vi "Go.vi"(9 "Timing Data":T1(array[cluster]), 10 "Control In":T2={"I-O.lvclass"=refnum, "Gantry"=refnum, "Dispenser"="COM1"}, 11 "Sensor Dispense in":refnum<class "Sensor Dispense.lvclass">) -> (2 "Control Out":T2={"I-O.lvclass"=refnum, "Gantry"=refnum, "Dispenser"="COM1"}, 3 "Sensor Dispense out":refnum<class "Sensor Dispense.lvclass">)   [LabVIEW 2021, in "Sensor Dispense.lvclass"]
uses:
  Sensor Dispense.lvclass
  C:/Users/HEP/Documents/GitHub/UCSB-Gantry-HEP/Classes/Routine/Dispense/Dispense.lvclass
  Classes/Controller/Controllers.ctl
  Classes/Controller/I-O/I-O.lvclass
  C:/Program Files (x86)/Aerotech/A3200/LabVIEW/2010/Bin/Aerotech.A3200.dll
  Program Files (x86)/Aerotech/A3200/LabVIEW/2010/Bin/Aerotech.A3200.dll
  Sensor Dispense.lvclass/Sensor Dispense.ctl
  Classes/Controller/Motion/Motion.lvclass
  Classes/Controller/Dispenser/Dispenser.lvclass
  Classes/Controller/Motion/A3200/A3200.lvclass
  Classes/Controller/Controller.lvclass
panel:
  out "error out":errorcluster
  in  "error in (no error)":errorcluster
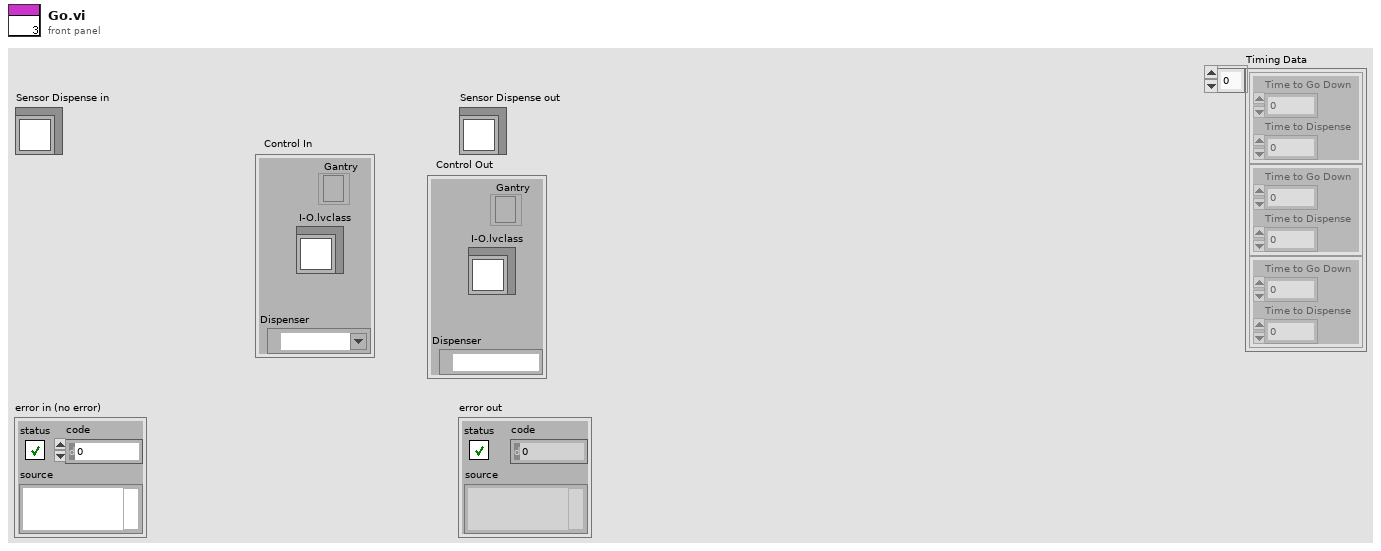
[diagram p1: front panel]
types:
  T1 = cluster{"Time to Go Down":i32, "Time to Dispense":i32}[]
  T2 = typedef "Controller.lvclass/Controllers.ctl" = cluster{"I-O.lvclass":refnum<class "I-O.lvclass">, "Gantry":refnum<k24>, "Dispenser":refnum<visa-resource-name>}
  T3 = cluster{"Endpoints":dbl[][], "Center":dbl[], "CW/CCW":dbl, "Dispense Type":enum16{"N-gon", "Square", "Arc", "Dot", "Line", "Circle"}}[]
  T4 = enum16{"N-gon", "Square", "Arc", "Dot", "Line", "Circle"}
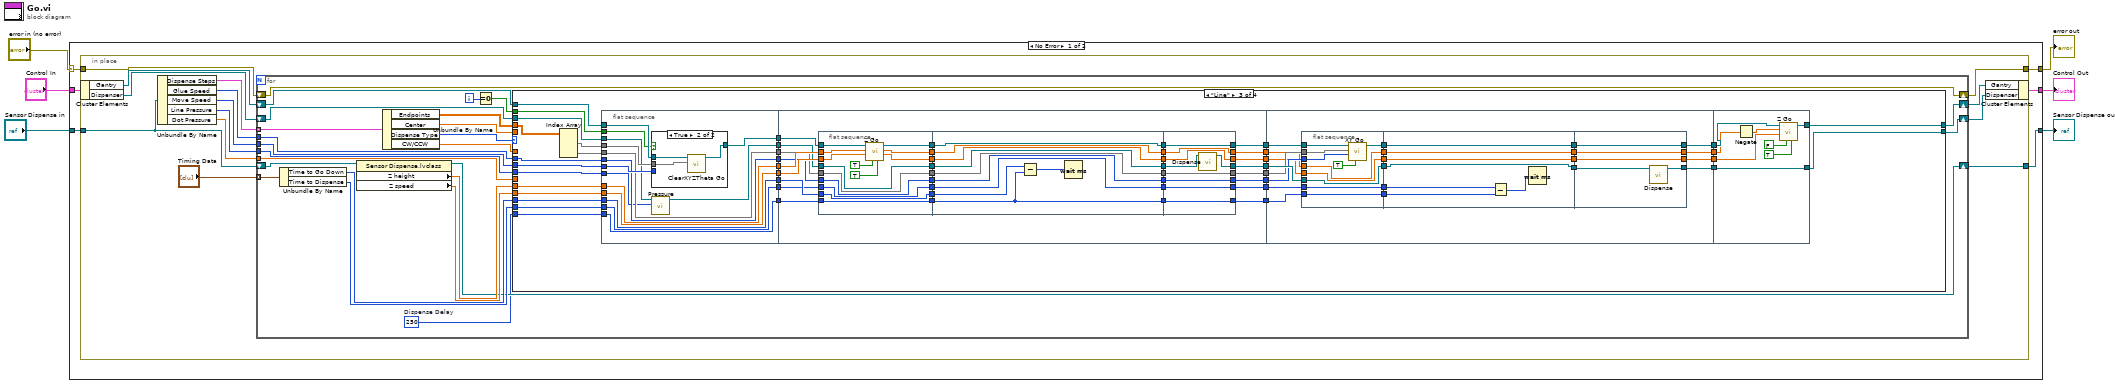
[diagram p0: block diagram]
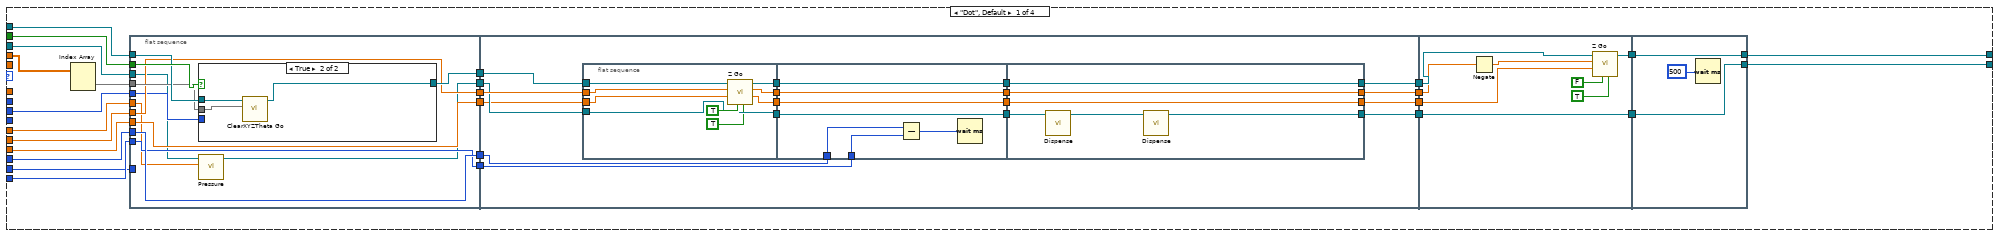
[diagram p2: hidden frame]
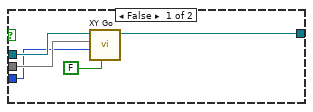
[diagram p3: hidden frame]
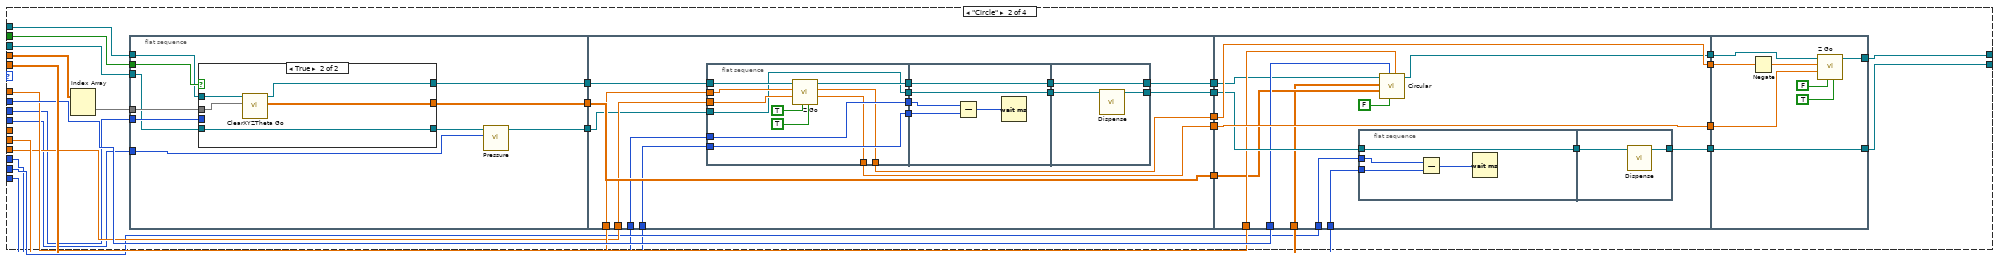
[diagram p4: hidden frame]
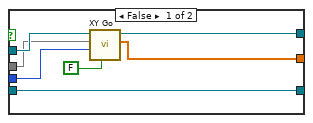
[diagram p5: hidden frame]
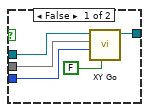
[diagram p6: hidden frame]
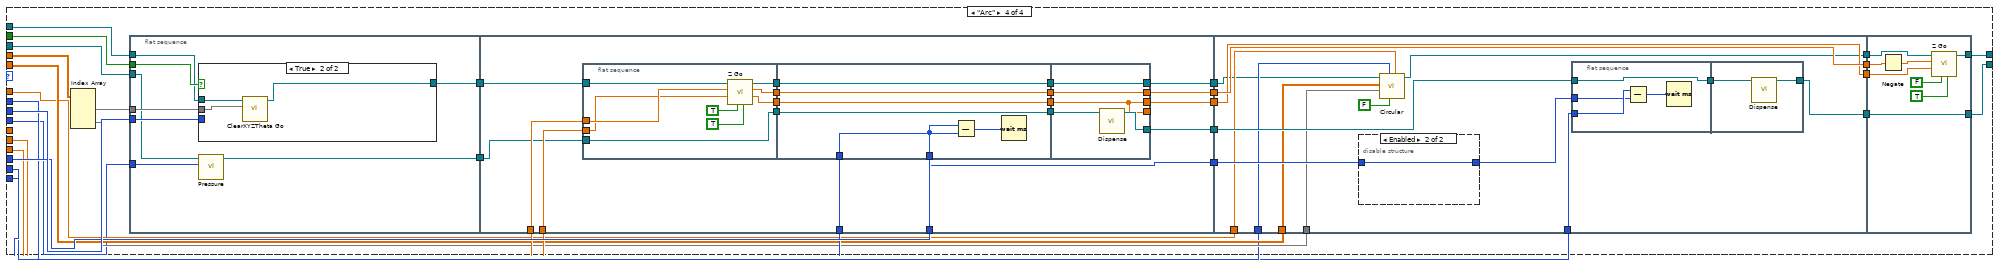
[diagram p7: hidden frame]
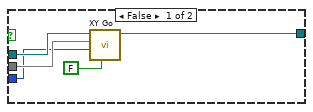
[diagram p8: hidden frame]
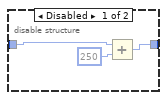
[diagram p9: hidden frame]
diagram:
  n1 = case shown="No Error" "error in (no error)" {
    selector: "error in (no error)" -> [w7 w562]
    tunnel: "Sensor Dispense in" -> [w12 w561]
    tunnel: [w11 w561] -> w5
    tunnel: "Control In" -> [w10 w560]
    tunnel: [w9 w560] -> w3
    tunnel: [w8 w562] -> w2
    frame No Error {
      n2 = in-place {
        in-place-border: w12 -> [w24]
        in-place-border: [w23] -> w11
        in-place-border: w7 -> [w17]
        in-place-border: [w16] -> w8
        n3 = in-place-cluster #1(w10) -> ("Gantry"=w25:refnum<k24>, "Dispenser"=w20:refnum<visa-resource-name>)
        n4 = Unbundle By Name(w24) -> ("Dispense Steps"=w21:T3, "Glue Speed"=w15:i32, "Move Speed"=w26:i32, "Line Pressure"=w13:i64, "Dot Pressure"=w14:dbl)
        n5 = for {
          tunnel: w26 -> [w50]
          shift-right: [w41] -> w22
          shift-left: w25 -> [w48]
          tunnel: w15 -> [w49]
          shift-right: [w32] -> w23
          shift-left: w24 -> [w46]
          tunnel: w21 -> [w43] mode=indexing
          shift-right: [w36] -> w18
          shift-left: w20 -> [w39]
          tunnel: "Timing Data" -> [w38] mode=indexing
          shift-right: [w27] -> w16
          shift-left: w17 -> [w27]
          tunnel: w14 -> [w29]
          tunnel: w13 -> [w28]
          i -> [w45]
          w31 = 250  # Dispense Delay
          n6 = Unbundle By Name(w38) -> ("Time to Go Down"=w37:i32, "Time to Dispense"=w33:i32)
          n7 = property class="Sensor Dispense.lvclass"(reference=w46) -> (reference out=w32:refnum<class "Sensor Dispense.lvclass">, "Z height"=w35:dbl, "Z speed"=w34:dbl)  [unwired: 1 in, 1 out]
          n8 = Unbundle By Name(w43) -> ("Endpoints"=w30:dbl[][], "Center"=w40:dbl[], "Dispense Type"=w42:T4, "CW/CCW"=w47:dbl)
          n9 = Equal To 0?(x=w45) -> (x = 0?=w44:bool)
          n10 = case shown="\"Line\"" w42 {
            tunnel: w40 -> [_ w172 _ w452]
            tunnel: w48 -> [w75 w173 w299 w461]
            tunnel: w50 -> [w58 w166 w298 w458]
            tunnel: [w74 w176 w295 w447] -> w41
            tunnel: w49 -> [_ w171 w285 w451]
            tunnel: w47 -> [_ w170 _ w450]
            tunnel: w34 -> [w66 w168 w282 w454]
            tunnel: w35 -> [w67 w169 w283 w455]
            tunnel: w44 -> [w76 w167 w297 w462]
            tunnel: w39 -> [w65 w150 w289 w443]
            tunnel: w37 -> [w63 w157 w287 w457]
            tunnel: w33 -> [w68 w158 w284 w449]
            tunnel: w31 -> [w69 w156 w288 w456]
            tunnel: [w73 w151 w292 w446] -> w36
            tunnel: w30 -> [w72 w155 w291 w460]
            tunnel: w29 -> [w57 _ _ _]
            tunnel: w28 -> [_ w148 w263 w442]
            frame "Dot", Default {
              n11 = Index Array(array=w72) -> (element=w71:dbl[])  [unwired: 2 in]
              n12 = flat-sequence {
                tunnel: w76 -> [w88]
                tunnel: w75 -> [w87]
                tunnel: w71 -> [w86]
                tunnel: [w85] -> w70
                tunnel: w69 -> [w82]
                tunnel: w68 -> [_]
                tunnel: w67 -> [w84]
                tunnel: w66 -> [w81]
                tunnel: w65 -> [w79]
                tunnel: [w84] -> w64
                tunnel: w63 -> [w83]
                tunnel: [w83] -> w62
                tunnel: [w82] -> w61
                tunnel: [w78] -> w60
                tunnel: [w81] -> w59
                tunnel: w58 -> [w80]
                tunnel: w57 -> [w77]
                tunnel: [w114] -> w54
                tunnel: w70 -> [w113]
                tunnel: [w110] -> w53
                tunnel: w64 -> [w109]
                tunnel: w62 -> [w108]
                tunnel: w61 -> [w107]
                tunnel: w60 -> [w106]
                tunnel: w59 -> [w103]
                tunnel: [w100] -> w52
                tunnel: [w99] -> w51
                tunnel: w54 -> [w142]
                tunnel: w53 -> [w141]
                tunnel: w52 -> [w140]
                tunnel: w51 -> [w139]
                tunnel: [w143] -> w56
                tunnel: [w142] -> w55
                tunnel: [w146] -> w73
                tunnel: [w147] -> w74
                tunnel: w56 -> [w147]
                tunnel: w55 -> [w146]
                frame #0 {
                  n13 = case shown="True" w88 {
                    tunnel: w87 -> [w93 w96]
                    tunnel: [w92 w95] -> w85
                    tunnel: w86 -> [w91 w94]
                    tunnel: w80 -> [w90 _]
                    frame False {
                      n14 = call "XY Go.vi"("return immediately"=FALSE, "Speed"=w90, "XY In"=w91, "Gantry In"=w93) -> ("Gantry Out"=w92:refnum<k24>)  [unwired: 5 in, 2 out]
                    }
                    frame True {
                      n15 = call "ClearXYZTheta Go.vi"("XYZTheta In"=w94, "Gantry In"=w96) -> ("Gantry Out"=w95:refnum<k24>)  [unwired: 7 in, 2 out]
                    }
                  }
                  n16 = call "Pressure.vi"("Pressure"=w77, "VISA resource name"=w79) -> ("VISA resource name out"=w78:refnum<visa-resource-name>)  [unwired: 8 in, 1 out]
                }
                frame #1 {
                  n17 = flat-sequence {
                    tunnel: w113 -> [w123]
                    tunnel: [w122] -> w111
                    tunnel: w109 -> [w121]
                    tunnel: w106 -> [w119]
                    tunnel: [w119] -> w105
                    tunnel: w103 -> [w118]
                    tunnel: [w117] -> w102
                    tunnel: [w116] -> w97
                    tunnel: [w129] -> w112
                    tunnel: w111 -> [w129]
                    tunnel: w108 -> [w128]
                    tunnel: w107 -> [w127]
                    tunnel: w105 -> [w126]
                    tunnel: [w126] -> w104
                    tunnel: w102 -> [w125]
                    tunnel: [w125] -> w101
                    tunnel: [w124] -> w98
                    tunnel: w97 -> [w124]
                    tunnel: [w136] -> w114
                    tunnel: w112 -> [w135]
                    tunnel: [w135] -> w110
                    tunnel: w104 -> [w134]
                    tunnel: w101 -> [w132]
                    tunnel: [w132] -> w100
                    tunnel: [w131] -> w99
                    tunnel: w98 -> [w131]
                    frame #0 {
                      n18 = call "Z Go.vi"("Increment"=TRUE, "Return Immediately"=TRUE, "Speed In"=w118, "Position In"=w121, "Gantry In"=w123) -> ("Speed Out"=w116:dbl, "Position Out"=w117:dbl, "Gantry Out"=w122:refnum<k24>)  [unwired: 3 in, 1 out]
                    }
                    frame #1 {
                      n19 = Subtract(x=w128, y=w127) -> (x-y=w130:i32)
                      n20 = Wait (ms)(milliseconds to wait=w130) -> ()  [unwired: 1 out]
                    }
                    frame #2 {
                      n21 = call "Dispense.vi"("Dispenser In"=w134) -> ("Dispenser Out"=w133:refnum<visa-resource-name>)  [unwired: 9 in, 1 out]
                      n22 = call "Dispense.vi"("Dispenser In"=w133) -> ("Dispenser Out"=w136:refnum<visa-resource-name>)  [unwired: 9 in, 1 out]
                    }
                  }
                }
                frame #2 {
                  n23 = Negate(x=w140) -> (-x=w144:dbl)
                  n24 = call "Z Go.vi"("Increment"=TRUE, "Return Immediately"=FALSE, "Speed In"=w139, "Position In"=w144, "Gantry In"=w141) -> ("Gantry Out"=w143:refnum<k24>)  [unwired: 3 in, 3 out]
                }
                frame #3 {
                  n25 = Wait (ms)(milliseconds to wait=u32 500) -> ()  [unwired: 1 out]
                }
              }
            }
            frame "Circle" {
              n26 = Index Array(array=w155) -> (element=w154:dbl[])  [unwired: 2 in]
              n27 = flat-sequence {
                tunnel: [w184] -> w175
                tunnel: w173 -> [w185]
                tunnel: w167 -> [w186]
                tunnel: w166 -> [w183]
                tunnel: [w182] -> w164
                tunnel: w154 -> [w181]
                tunnel: w150 -> [w180]
                tunnel: [w178] -> w149
                tunnel: w148 -> [w177]
                tunnel: w169 -> [w208]
                tunnel: w168 -> [w209]
                tunnel: [w215] -> w165
                tunnel: [w206] -> w163
                tunnel: [w207] -> w162
                tunnel: w164 -> [w215]
                tunnel: w175 -> [w205]
                tunnel: [w214] -> w159
                tunnel: w157 -> [w213]
                tunnel: w156 -> [w212]
                tunnel: [w202] -> w153
                tunnel: w149 -> [w201]
                tunnel: [w235] -> w174
                tunnel: [w248] -> w161
                tunnel: [w247] -> w160
                tunnel: w156 -> [w245]
                tunnel: w158 -> [w246]
                tunnel: w159 -> [w243]
                tunnel: w165 -> [w238]
                tunnel: w163 -> [w248]
                tunnel: w162 -> [w247]
                tunnel: w170 -> [w241]
                tunnel: w171 -> [w239]
                tunnel: w172 -> [w237]
                tunnel: w153 -> [w236]
                tunnel: [w244] -> w152
                tunnel: [w260] -> w176
                tunnel: w174 -> [w261]
                tunnel: w161 -> [w262]
                tunnel: w160 -> [w259]
                tunnel: w152 -> [w258]
                tunnel: [w258] -> w151
                frame #0 {
                  n28 = case shown="True" w186 {
                    tunnel: w185 -> [w193 w198]
                    tunnel: [w192 w197] -> w184
                    tunnel: w183 -> [w191 _]
                    tunnel: [w190 w195] -> w182
                    tunnel: w181 -> [w189 w196]
                    tunnel: w180 -> [w188 w194]
                    tunnel: [w188 w194] -> w179
                    frame False {
                      n29 = call "XY Go.vi"("return immediately"=FALSE, "Speed"=w191, "XY In"=w189, "Gantry In"=w193) -> ("XY Out"=w190:dbl[], "Gantry Out"=w192:refnum<k24>)  [unwired: 5 in, 1 out]
                    }
                    frame True {
                      n30 = call "ClearXYZTheta Go.vi"("XYZTheta In"=w196, "Gantry In"=w198) -> ("XYZTheta Out"=w195:dbl[], "Gantry Out"=w197:refnum<k24>)  [unwired: 7 in, 1 out]
                    }
                  }
                  n31 = call "Pressure.vi"("Pressure"=w177, "VISA resource name"=w179) -> ("VISA resource name out"=w178:refnum<visa-resource-name>)  [unwired: 8 in, 1 out]
                }
                frame #1 {
                  n32 = flat-sequence {
                    tunnel: w212 -> [w225]
                    tunnel: w213 -> [w226]
                    tunnel: [w226] -> w211
                    tunnel: [w225] -> w210
                    tunnel: w209 -> [w224]
                    tunnel: w208 -> [w223]
                    tunnel: [w222] -> w207
                    tunnel: [w221] -> w206
                    tunnel: w205 -> [w220]
                    tunnel: [w219] -> w204
                    tunnel: w201 -> [w217]
                    tunnel: [w217] -> w200
                    tunnel: w211 -> [w230]
                    tunnel: w210 -> [w229]
                    tunnel: w204 -> [w228]
                    tunnel: [w228] -> w203
                    tunnel: w200 -> [w227]
                    tunnel: [w227] -> w199
                    tunnel: [w234] -> w214
                    tunnel: w203 -> [w233]
                    tunnel: [w233] -> w202
                    tunnel: w199 -> [w232]
                    frame #0 {
                      n33 = call "Z Go.vi"("Increment"=TRUE, "Return Immediately"=TRUE ("return immediately"), "Speed In"=w224, "Position In"=w223, "Gantry In"=w220) -> ("Speed Out"=w222:dbl, "Position Out"=w221:dbl, "Gantry Out"=w219:refnum<k24>)  [unwired: 3 in, 1 out]
                    }
                    frame #1 {
                      n34 = Subtract(x=w230, y=w229) -> (x-y=w231:i32)
                      n35 = Wait (ms)(milliseconds to wait=w231) -> ()  [unwired: 1 out]
                    }
                    frame #2 {
                      n36 = call "Dispense.vi"("Dispenser In"=w232) -> ("Dispenser Out"=w234:refnum<visa-resource-name>)  [unwired: 9 in, 1 out]
                    }
                  }
                }
                frame #2 {
                  n37 = flat-sequence {
                    tunnel: [w249] -> w242
                    tunnel: w246 -> [w252]
                    tunnel: w245 -> [w251]
                    tunnel: w243 -> [w249]
                    tunnel: [w254] -> w244
                    tunnel: w242 -> [w253]
                    frame #0 {
                      n38 = Subtract(x=w252, y=w251) -> (x-y=w250:i32)
                      n39 = Wait (ms)(milliseconds to wait=w250) -> ()  [unwired: 1 out]
                    }
                    frame #1 {
                      n40 = call "Dispense.vi"("Dispenser In"=w253) -> ("Dispenser Out"=w254:refnum<visa-resource-name>)  [unwired: 9 in, 1 out]
                    }
                  }
                  n41 = call "Circular.vi"("Direction"=w241, "return immediately"=FALSE, "Speed"=w239, "XY End"=w238, "XY Center"=w237, "Gantry In"=w236) -> ("Gantry Out"=w235:refnum<k24>)  [unwired: 4 in, 1 out]
                }
                frame #3 {
                  n42 = Negate(x=w262) -> (-x=w257:dbl)
                  n43 = call "Z Go.vi"("Increment"=TRUE, "Return Immediately"=FALSE, "Speed In"=w259, "Position In"=w257, "Gantry In"=w261) -> ("Gantry Out"=w260:refnum<k24>)  [unwired: 3 in, 3 out]
                }
              }
            }
            frame "Line" {
              n44 = Index Array(array=w291) -> (element #1=w290:dbl[], element #2=w286:dbl[])  [unwired: 4 in]
              n45 = flat-sequence {
                tunnel: w299 -> [w314]
                tunnel: w298 -> [w313]
                tunnel: w297 -> [w312]
                tunnel: [w311] -> w296
                tunnel: w290 -> [w310]
                tunnel: w289 -> [w302]
                tunnel: w288 -> [w306]
                tunnel: w287 -> [w307]
                tunnel: w286 -> [w305]
                tunnel: w285 -> [w304]
                tunnel: w284 -> [w303]
                tunnel: w283 -> [w309]
                tunnel: w282 -> [w308]
                tunnel: [w309] -> w281
                tunnel: [w308] -> w280
                tunnel: [w307] -> w278
                tunnel: [w306] -> w277
                tunnel: [w301] -> w276
                tunnel: [w305] -> w274
                tunnel: [w304] -> w272
                tunnel: [w303] -> w270
                tunnel: w263 -> [w300]
                tunnel: w296 -> [w355]
                tunnel: [w356] -> w294
                tunnel: w281 -> [w354]
                tunnel: w280 -> [w353]
                tunnel: [w350] -> w279
                tunnel: w278 -> [w348]
                tunnel: w277 -> [w346]
                tunnel: w276 -> [w343]
                tunnel: [w342] -> w275
                tunnel: w274 -> [w339]
                tunnel: [w338] -> w273
                tunnel: w272 -> [w335]
                tunnel: [w331] -> w271
                tunnel: w270 -> [w332]
                tunnel: [w330] -> w269
                tunnel: [w328] -> w266
                tunnel: [w325] -> w264
                tunnel: w294 -> [w407]
                tunnel: [w411] -> w293
                tunnel: w279 -> [w410]
                tunnel: w275 -> [w406]
                tunnel: w273 -> [w405]
                tunnel: w271 -> [w402]
                tunnel: w269 -> [w400]
                tunnel: [w398] -> w268
                tunnel: [w397] -> w267
                tunnel: w266 -> [w394]
                tunnel: [w393] -> w265
                tunnel: w264 -> [w390]
                tunnel: [w441] -> w295
                tunnel: w293 -> [w440]
                tunnel: [w440] -> w292
                tunnel: w268 -> [w439]
                tunnel: w267 -> [w438]
                tunnel: w265 -> [w436]
                frame #0 {
                  n46 = case shown="True" w312 {
                    tunnel: w314 -> [w319 w322]
                    tunnel: w313 -> [w318 _]
                    tunnel: [w317 w321] -> w311
                    tunnel: w310 -> [w316 w320]
                    frame False {
                      n47 = call "XY Go.vi"("return immediately"=FALSE, "Speed"=w318, "XY In"=w316, "Gantry In"=w319) -> ("Gantry Out"=w317:refnum<k24>)  [unwired: 5 in, 2 out]
                    }
                    frame True {
                      n48 = call "ClearXYZTheta Go.vi"("XYZTheta In"=w320, "Gantry In"=w322) -> ("Gantry Out"=w321:refnum<k24>)  [unwired: 7 in, 2 out]
                    }
                  }
                  n49 = call "Pressure.vi"("Pressure"=w300, "VISA resource name"=w302) -> ("VISA resource name out"=w301:refnum<visa-resource-name>)  [unwired: 8 in, 1 out]
                }
                frame #1 {
                  n50 = flat-sequence {
                    tunnel: w355 -> [w370]
                    tunnel: w354 -> [w369]
                    tunnel: w353 -> [w368]
                    tunnel: [w366] -> w352
                    tunnel: [w365] -> w349
                    tunnel: w348 -> [w365]
                    tunnel: [w364] -> w347
                    tunnel: w346 -> [w364]
                    tunnel: [w363] -> w344
                    tunnel: w343 -> [w363]
                    tunnel: [w362] -> w340
                    tunnel: w339 -> [w362]
                    tunnel: [w361] -> w336
                    tunnel: w335 -> [w361]
                    tunnel: [w360] -> w333
                    tunnel: w332 -> [w360]
                    tunnel: [w359] -> w326
                    tunnel: [w358] -> w323
                    tunnel: w352 -> [w379]
                    tunnel: [w379] -> w351
                    tunnel: w349 -> [w378]
                    tunnel: w347 -> [w373]
                    tunnel: [w377] -> w345
                    tunnel: w344 -> [w377]
                    tunnel: [w376] -> w341
                    tunnel: w340 -> [w376]
                    tunnel: [w375] -> w337
                    tunnel: w336 -> [w375]
                    tunnel: [w374] -> w334
                    tunnel: w333 -> [w374]
                    tunnel: [w373] -> w329
                    tunnel: [w372] -> w327
                    tunnel: w326 -> [w372]
                    tunnel: [w371] -> w324
                    tunnel: w323 -> [w371]
                    tunnel: [w389] -> w356
                    tunnel: w351 -> [w388]
                    tunnel: [w388] -> w350
                    tunnel: w345 -> [w383]
                    tunnel: [w387] -> w342
                    tunnel: w341 -> [w387]
                    tunnel: [w386] -> w338
                    tunnel: w337 -> [w386]
                    tunnel: w334 -> [w385]
                    tunnel: [w385] -> w331
                    tunnel: [w384] -> w330
                    tunnel: w329 -> [w384]
                    tunnel: [w382] -> w328
                    tunnel: w327 -> [w382]
                    tunnel: [w381] -> w325
                    tunnel: w324 -> [w381]
                    frame #0 {
                      n51 = call "Z Go.vi"("Increment"=TRUE, "Return Immediately"=TRUE, "Speed In"=w368, "Position In"=w369, "Gantry In"=w370) -> ("Speed Out"=w358:dbl, "Position Out"=w359:dbl, "Gantry Out"=w366:refnum<k24>)  [unwired: 3 in, 1 out]
                    }
                    frame #1 {
                      n52 = Subtract(x=w378, y=w373) -> (x-y=w380:i32)
                      n53 = Wait (ms)(milliseconds to wait=w380) -> ()  [unwired: 1 out]
                    }
                    frame #2 {
                      n54 = call "Dispense.vi"("Dispenser In"=w383) -> ("Dispenser Out"=w389:refnum<visa-resource-name>)  [unwired: 9 in, 1 out]
                    }
                  }
                }
                frame #2 {
                  n55 = flat-sequence {
                    tunnel: w410 -> [w420]
                    tunnel: [w419] -> w408
                    tunnel: w407 -> [w419]
                    tunnel: w406 -> [w418]
                    tunnel: w405 -> [w417]
                    tunnel: [w416] -> w404
                    tunnel: [w415] -> w403
                    tunnel: w402 -> [w415]
                    tunnel: [w414] -> w401
                    tunnel: w400 -> [w414]
                    tunnel: [w413] -> w395
                    tunnel: w394 -> [w413]
                    tunnel: [w412] -> w391
                    tunnel: w390 -> [w412]
                    tunnel: [w427] -> w409
                    tunnel: w408 -> [w427]
                    tunnel: w404 -> [w424]
                    tunnel: w403 -> [w426]
                    tunnel: w401 -> [w425]
                    tunnel: [w424] -> w399
                    tunnel: [w423] -> w396
                    tunnel: w395 -> [w423]
                    tunnel: [w422] -> w392
                    tunnel: w391 -> [w422]
                    tunnel: [w433] -> w411
                    tunnel: w409 -> [w431]
                    tunnel: w399 -> [w432]
                    tunnel: [w432] -> w398
                    tunnel: [w430] -> w397
                    tunnel: w396 -> [w430]
                    tunnel: [w429] -> w393
                    tunnel: w392 -> [w429]
                    frame #0 {
                      n56 = call "XY Go.vi"("return immediately"=TRUE, "Speed"=w417, "XY In"=w418, "Gantry In"=w420) -> ("Gantry Out"=w416:refnum<k24>)  [unwired: 5 in, 2 out]
                    }
                    frame #1 {
                      n57 = Subtract(x=w426, y=w425) -> (x-y=w428:i32)
                      n58 = Wait (ms)(milliseconds to wait=w428) -> ()  [unwired: 1 out]
                    }
                    frame #2 {
                      n59 = call "Dispense.vi"("Dispenser In"=w431) -> ("Dispenser Out"=w433:refnum<visa-resource-name>)  [unwired: 9 in, 1 out]
                    }
                  }
                }
                frame #3 {
                  n60 = Negate(x=w438) -> (-x=w437:dbl)
                  n61 = call "Z Go.vi"("Increment"=TRUE, "Return Immediately"=FALSE, "Speed In"=w436, "Position In"=w437, "Gantry In"=w439) -> ("Gantry Out"=w441:refnum<k24>)  [unwired: 3 in, 3 out]
                }
              }
            }
            frame "Arc" {
              n62 = Index Array(array=w460) -> (element #1=w459:dbl[], element #2=w453:dbl[])  [unwired: 4 in]
              n63 = flat-sequence {
                tunnel: [w478] -> w470
                tunnel: w462 -> [w477]
                tunnel: w461 -> [w476]
                tunnel: w459 -> [w475]
                tunnel: w458 -> [w474]
                tunnel: [w473] -> w444
                tunnel: w443 -> [w472]
                tunnel: w442 -> [w471]
                tunnel: w470 -> [w504]
                tunnel: [w505] -> w469
                tunnel: [w501] -> w468
                tunnel: [w498] -> w467
                tunnel: [w495] -> w466
                tunnel: w457 -> [w494]
                tunnel: w456 -> [w493]
                tunnel: w455 -> [w492]
                tunnel: w454 -> [w491]
                tunnel: [w490] -> w448
                tunnel: w444 -> [w489]
                tunnel: w469 -> [w535]
                tunnel: [w538] -> w465
                tunnel: w468 -> [w528]
                tunnel: w467 -> [w541]
                tunnel: [w541] -> w464
                tunnel: w466 -> [w540]
                tunnel: [w540] -> w463
                tunnel: w453 -> [w530]
                tunnel: w452 -> [w529]
                tunnel: w451 -> [w531]
                tunnel: w450 -> [w533]
                tunnel: w449 -> [w539]
                tunnel: w448 -> [w537]
                tunnel: [w527] -> w445
                tunnel: [w559] -> w447
                tunnel: w465 -> [w558]
                tunnel: [w558] -> w446
                tunnel: w464 -> [w556]
                tunnel: w463 -> [w554]
                tunnel: w445 -> [w557]
                frame #0 {
                  n64 = case shown="True" w477 {
                    tunnel: [w483 w486] -> w478
                    tunnel: w476 -> [w482 w485]
                    tunnel: w475 -> [w481 w484]
                    tunnel: w474 -> [w480 _]
                    frame False {
                      n65 = call "XY Go.vi"("return immediately"=FALSE, "Speed"=w480, "XY In"=w481, "Gantry In"=w482) -> ("Gantry Out"=w483:refnum<k24>)  [unwired: 5 in, 2 out]
                    }
                    frame True {
                      n66 = call "ClearXYZTheta Go.vi"("XYZTheta In"=w484, "Gantry In"=w485) -> ("Gantry Out"=w486:refnum<k24>)  [unwired: 7 in, 2 out]
                    }
                  }
                  n67 = call "Pressure.vi"("Pressure"=w471, "VISA resource name"=w472) -> ("VISA resource name out"=w473:refnum<visa-resource-name>)  [unwired: 8 in, 1 out]
                }
                frame #1 {
                  n68 = flat-sequence {
                    tunnel: w504 -> [w514]
                    tunnel: [w512] -> w503
                    tunnel: [w511] -> w500
                    tunnel: [w510] -> w499
                    tunnel: w492 -> [w509]
                    tunnel: w491 -> [w508]
                    tunnel: w489 -> [w506]
                    tunnel: [w506] -> w488
                    tunnel: w503 -> [w520]
                    tunnel: [w520] -> w502
                    tunnel: w500 -> [w519]
                    tunnel: w499 -> [w518]
                    tunnel: [w519] -> w497
                    tunnel: [w518] -> w496
                    tunnel: w494 -> [w517]
                    tunnel: w493 -> [w516]
                    tunnel: [w516] -> w490
                    tunnel: w488 -> [w515]
                    tunnel: [w515] -> w487
                    tunnel: [w526] -> w505
                    tunnel: w502 -> [w525]
                    tunnel: [w525] -> w501
                    tunnel: [w524] -> w498
                    tunnel: w497 -> [w524]
                    tunnel: w496 -> [w523]
                    tunnel: [w523] -> _
                    tunnel: [w523] -> w495
                    tunnel: w487 -> [w522]
                    frame #0 {
                      n69 = call "Z Go.vi"("Increment"=TRUE, "Return Immediately"=TRUE, "Speed In"=w508, "Position In"=w509, "Gantry In"=w514) -> ("Speed Out"=w510:dbl, "Position Out"=w511:dbl, "Gantry Out"=w512:refnum<k24>)  [unwired: 3 in, 1 out]
                    }
                    frame #1 {
                      n70 = Subtract(x=w517, y=w516) -> (x-y=w521:i32)
                      n71 = Wait (ms)(milliseconds to wait=w521) -> ()  [unwired: 1 out]
                    }
                    frame #2 {
                      n72 = call "Dispense.vi"("Dispenser In"=w522) -> ("Dispenser Out"=w526:refnum<visa-resource-name>)  [unwired: 9 in, 1 out]
                    }
                  }
                }
                frame #2 {
                  n73 = disable-structure shown="Enabled" {
                    disable-tunnel: w537 -> [w544 w545]
                    disable-tunnel: [w542 w545] -> w536
                    frame Disabled {
                      n74 = Add(x=w544, y=250) -> (x+y=w542:i32)
                    }
                    frame Enabled {
                    }
                  }
                  n75 = call "Circular.vi"("Direction"=w533, "return immediately"=FALSE, "Speed"=w531, "XY End"=w530, "XY Center"=w529, "Gantry In"=w528) -> ("Gantry Out"=w527:refnum<k24>)  [unwired: 4 in, 1 out]
                  n76 = flat-sequence {
                    tunnel: [w546] -> w534
                    tunnel: w539 -> [w549]
                    tunnel: w536 -> [w548]
                    tunnel: w535 -> [w546]
                    tunnel: [w551] -> w538
                    tunnel: w534 -> [w550]
                    frame #0 {
                      n77 = Subtract(x=w549, y=w548) -> (x-y=w547:i32)
                      n78 = Wait (ms)(milliseconds to wait=w547) -> ()  [unwired: 1 out]
                    }
                    frame #1 {
                      n79 = call "Dispense.vi"("Dispenser In"=w550) -> ("Dispenser Out"=w551:refnum<visa-resource-name>)  [unwired: 9 in, 1 out]
                    }
                  }
                }
                frame #3 {
                  n80 = Negate(x=w556) -> (-x=w555:dbl)
                  n81 = call "Z Go.vi"("Increment"=TRUE, "Return Immediately"=FALSE, "Speed In"=w554, "Position In"=w555, "Gantry In"=w557) -> ("Gantry Out"=w559:refnum<k24>)  [unwired: 3 in, 3 out]
                }
              }
            }
          }
        }
        n82 = in-place-cluster #1("Gantry"=w22, "Dispenser"=w18) -> (w9:T2)
      }
    }
    frame Error {
    }
  }
  "error out" <- w2
  "Sensor Dispense out" <- w5
  "Control Out" <- w3
